vi "optos_indexing_v2.vi"(11 "Array in":bool[](array[boolean])) -> (3 "Array  out":bool[](array[boolean]))   [LabVIEW 2018, in "MB Relay.lvlib"]
uses:
  MB Relay.lvlib
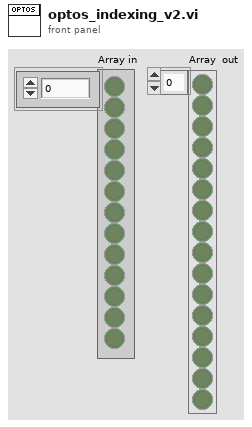
[diagram p1: front panel]
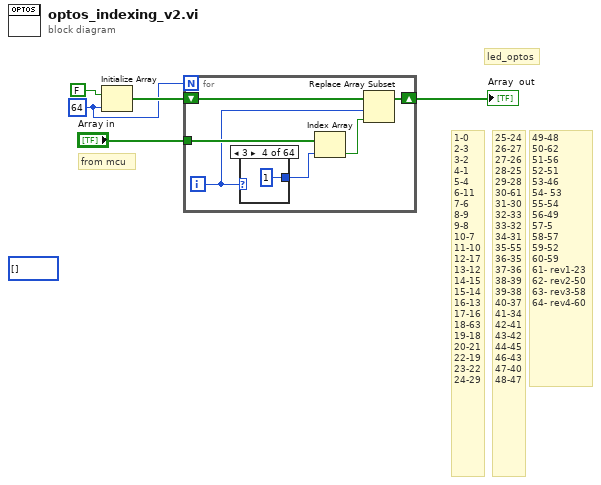
[diagram p0: block diagram]
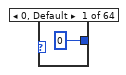
[diagram p2: hidden frame]
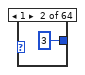
[diagram p3: hidden frame]
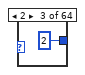
[diagram p4: hidden frame]
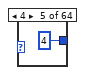
[diagram p5: hidden frame]
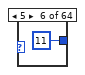
[diagram p6: hidden frame]
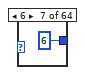
[diagram p7: hidden frame]
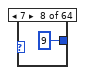
[diagram p8: hidden frame]
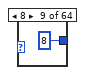
[diagram p9: hidden frame]
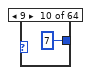
[diagram p10: hidden frame]
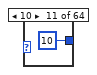
[diagram p11: hidden frame]
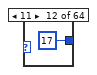
[diagram p12: hidden frame]
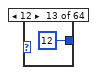
[diagram p13: hidden frame]
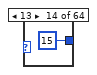
[diagram p14: hidden frame]
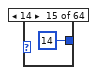
[diagram p15: hidden frame]
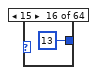
[diagram p16: hidden frame]
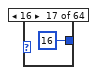
[diagram p17: hidden frame]
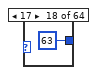
[diagram p18: hidden frame]
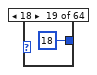
[diagram p19: hidden frame]
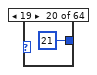
[diagram p20: hidden frame]
diagram:
  (unwired) i32[] []
  w1 = 64 ("dimension size")
  # "49-48\n50-62\n51-56\n52-51\n53-46\n54- 53\n55-54\n56-49\n57-5\n58-57\n59-52\n60-59\n61- rev1-23\n62- rev2-50\n63- rev3-58\n64- rev4-60"
  # "25-24\n26-27\n27-26\n28-25\n29-28\n30-61\n31-30\n32-33\n33-32\n34-31\n35-55\n36-35\n37-36\n38-39\n39-38\n40-37\n41-34\n42-41\n43-42\n44-45\n46-43\n47-40\n48-47"
  # "from mcu"
  # "led_optos"
  # "1-0\n2-3\n3-2\n4-1\n5-4\n6-11\n7-6\n8-9\n9-8\n10-7\n11-10\n12-17\n13-12\n14-15\n15-14\n16-13\n17-16\n18-63\n19-18\n20-21\n22-19\n23-22\n24-29"
  n1 = Initialize Array(FALSE, w1) -> (w4:bool[])
  n2 = for {
    N: w1 -> [_]
    tunnel: "Array in" -> [w11]
    shift-right: [w6] -> w2
    shift-left: w4 -> [w9]
    i -> [w8]
    n3 = case shown="3" w8 {
      tunnel: [0 3 2 1 4 11 6 9 8 7 10 17 12 15 14 13 16 63 18 21 20 19 22 29 24 27 26 25 28 61 30 33 32 31 55 35 36 39 38 37 34 41 42 45 44 43 40 47 48 62 56 51 46 53 54 49 5 57 52 59 23 50 58 60] -> w10
      frame 0, Default {
      }
      frame 1 {
      }
      frame 2 {
      }
      frame 3 {
      }
      frame 4 {
      }
      frame 5 {
      }
      frame 6 {
      }
      frame 7 {
      }
      frame 8 {
      }
      frame 9 {
      }
      frame 10 {
      }
      frame 11 {
      }
      frame 12 {
      }
      frame 13 {
      }
      frame 14 {
      }
      frame 15 {
      }
      frame 16 {
      }
      frame 17 {
      }
      frame 18 {
      }
      frame 19 {
      }
      frame 20 {
      }
      frame 21 {
      }
      frame 22 {
      }
      frame 23 {
      }
      frame 24 {
      }
      frame 25 {
      }
      frame 26 {
      }
      frame 27 {
      }
      frame 28 {
      }
      frame 29 {
      }
      frame 30 {
      }
      frame 31 {
      }
      frame 32 {
      }
      frame 33 {
      }
      frame 34 {
      }
      frame 35 {
      }
      frame 36 {
      }
      frame 37 {
      }
      frame 38 {
      }
      frame 39 {
      }
      frame 40 {
      }
      frame 41 {
      }
      frame 42 {
      }
      frame 43 {
      }
      frame 44 {
      }
      frame 45 {
      }
      frame 46 {
      }
      frame 47 {
      }
      frame 48 {
      }
      frame 49 {
      }
      frame 50 {
      }
      frame 51 {
      }
      frame 52 {
      }
      frame 53 {
      }
      frame 54 {
      }
      frame 55 {
      }
      frame 56 {
      }
      frame 57 {
      }
      frame 58 {
      }
      frame 59 {
      }
      frame 60 {
      }
      frame 61 {
      }
      frame 62 {
      }
      frame 63 {
      }
    }
    n4 = Index Array(array=w11, index=w10) -> (element=w7:bool)
    n5 = Replace Array Subset(array=w9, new element=w7, index=w8) -> (w6:bool[])
  }
  "Array  out" <- w2
